vi "DQMH Load API Tester.vi"(7 "Application reference":refnum<vi>, 8 "error in (no error)":errorcluster, 10 "Module Name":string, 11 "Path to module directory":path) -> (0 "error out":errorcluster)   [LabVIEW 2014, in "hse-dqmh-dynamicrequesters.lvlib"]
doc: "Calls the \"Load Module\" request VI of the module in <b>path</b>\n\n____\nHAMPEL SOFTWARE ENGINEERING v0.7.0 (2018-07-16 18:12)"
uses:
  hse-dqmh-dynamicrequesters.lvlib
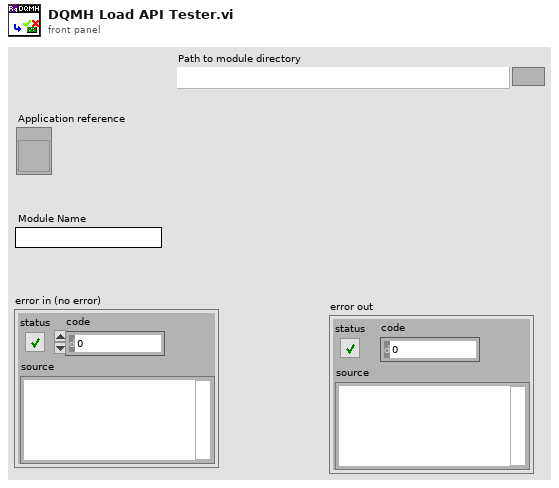
[diagram p1: front panel]
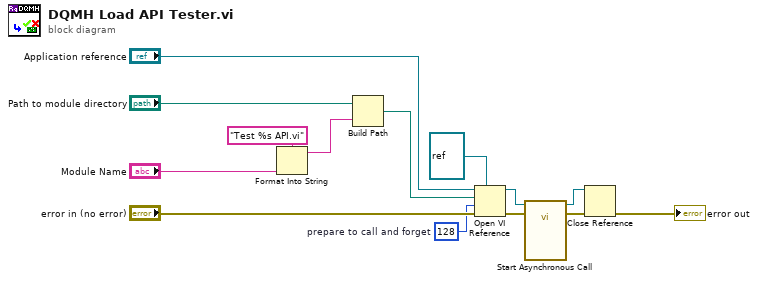
[diagram p0: block diagram]
diagram:
  w8 = 128  # prepare to call and forget
  n1 = Format Into String(format string="Test %s API.vi" ("name or relative path"), "Module Name") -> (resulting string=w6:string)  [unwired: 2 in, 1 out]
  n2 = Build Path(base path="Path to module directory", name or relative path=w6) -> (appended path=w10:path)
  n3 = Open VI Reference(type specifier VI Refnum (for type only)=refnum<vi> refnum, application reference (local)="Application reference", vi path=w10, options=w8, error in (no error)="error in (no error)") -> (vi reference=w2:refnum<vi>, error out=w4:errorcluster)  [unwired: 1 in]
  n4 = call-by-ref "Start Asynchronous Call"(reference=w2, error in=w4) -> (reference out=w1:refnum<vi>, error out=w3:errorcluster)  [unwired: 12 in]
  n5 = Close Reference(reference=w1, error in (no error)=w3) -> (error out=→"error out":errorcluster)
